vi "RT_tst.vi"() -> ()   [LabVIEW 2011]
uses:
  <vilib>/platform/TimedLoop/XDataNode/XDataNode.xnode
  <vilib>/Platform/TimedLoop/XDataNode/nitl_modes.ctl
  <vilib>/Platform/TimedLoop/XDataNode/XDNodeRunTimeDep.lvlib
  <vilib>/Platform/TimedLoop/XDataNode/wakeup.ctl
  <vilib>/Platform/TimedLoop/XDataNode/timing_clust.ctl
panel:
  out "Numeric":dbl
  out "Waveform Chart":dbl(graph)
  in  "stop":bool
  out "Iteration Duration":i64
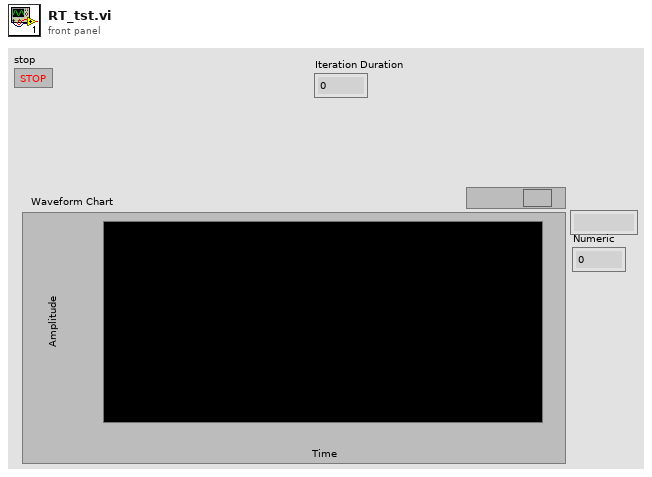
[diagram p1: front panel]
types:
  T1 = typedef "XDNodeRunTimeDep.lvlib/timing_clust.ctl" = cluster{"Expected End [f-1]":u64, "Actual End [f-1]":u64, "Finished Late? [f-1]":bool, "Expected End [i-1]":u64, "Actual End [i-1]":u64, "Finished Late? [i-1]":bool, "Expected Start [i]":u64, "Actual Start [i]":u64, "Expected Start [f]":u64, "Actual Start [f]":u64, "Source Name":string, "Structure Name":string, "Period":i64, "Deadline":i64, "Offset":i64, "Start":i64, "Priority":i32, "Timeout":i32, "Mode":T2, "Wakeup Reason":T3, "Error":errorcluster, "Source Type":string, "Secondary Source Type":string, "Global End Time":u64, "Global Start Time":u64, "Frame Duration":u64, "Iteration Duration":u64, "Assigned CPU":i32, "I/O Scan Engine Mode":u32}
  T2 = typedef "XDNodeRunTimeDep.lvlib/nitl_modes.ctl" = enum32{"No Change", "Process missed periods, maintain original phase", "Discard missed periods, maintain original phase", "Process missed periods, ignore original phase", "Discard missed periods, ignore original phase"}
  T3 = typedef "XDNodeRunTimeDep.lvlib/wakeup.ctl" = enum32{"Normal", "Aborted", "Asynchronous wakeup", "Timing source error", "Timed loop error", "Timeout"}
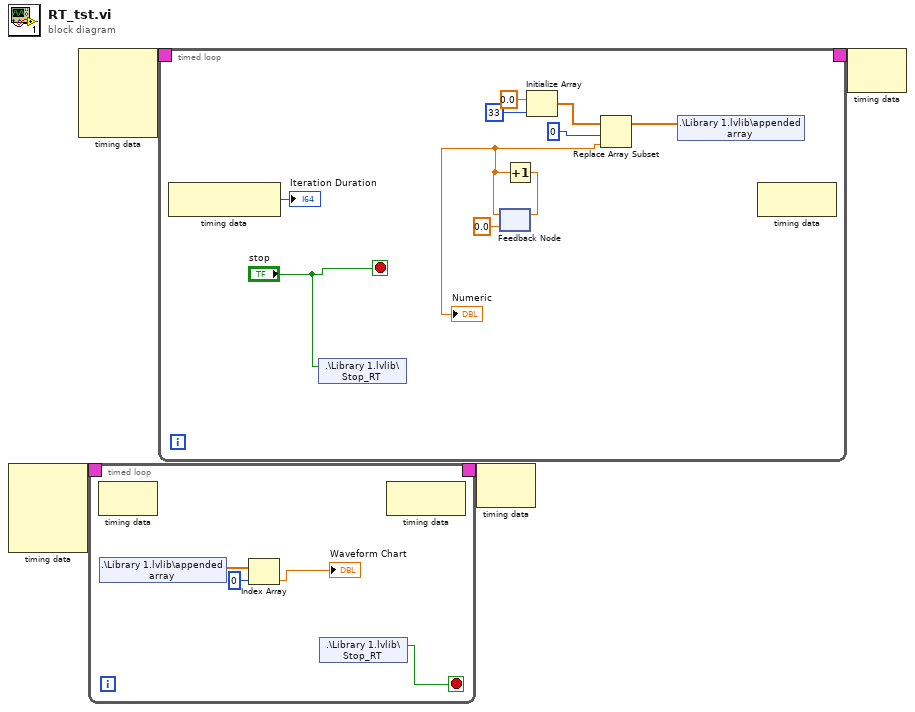
[diagram p0: block diagram]
diagram:
  n1 = node-c288() -> (w2:T1)  [unwired: 4 in]
  n2 = node-c288() -> (w4:T1)  [unwired: 4 in]
  n3 = timed-loop {
    timing: w2 -> [_]
    timing-out: [_] -> w1
    stop <- w5 stop-if-true
    n4 = node-c288() -> ()  [unwired: 1 in, 1 out]
    n5 = shared-variable ".\\Library 1.lvlib\\appended array"() -> (w8:dbl[])  [unwired: 1 in, 1 out]
    n6 = Index Array(array=w8, index=0) -> (element=→"Waveform Chart":dbl)
    n7 = shared-variable ".\\Library 1.lvlib\\Stop_RT"() -> (w5:bool)  [unwired: 1 in, 1 out]
    n8 = node-c288() -> ()  [unwired: 1 in, 1 out]
  }
  n9 = timed-loop {
    timing: w4 -> [_]
    timing-out: [_] -> w3
    stop <- "stop" stop-if-true
    n10 = node-c288() -> (→"Iteration Duration":i64)  [unwired: 1 in]
    n11 = shared-variable ".\\Library 1.lvlib\\Stop_RT"("stop") -> ()  [unwired: 1 in, 1 out]
    n12 = feedback #1(0.0) -> (w13:dbl)
    "Numeric" <- w13
    n13 = Increment(x=w13) -> (x+1=w19:dbl)
    n14 = feedback-in #1(w19) -> ()
    n15 = Initialize Array(0.0 ("element"), 33 ("dimension size")) -> (w16:dbl[])
    n16 = Replace Array Subset(array=w16, new element=w13, index=0) -> (w15:dbl[])
    n17 = shared-variable ".\\Library 1.lvlib\\appended array"(w15) -> ()  [unwired: 1 in, 1 out]
    n18 = node-c288() -> ()  [unwired: 1 in, 1 out]
  }
  n19 = node-c288(w1) -> ()  [unwired: 1 out]
  n20 = node-c288(w3) -> ()  [unwired: 1 out]
